vi "MMI GetAsyncKeyState.vi"(6 "Enum":T1(ring), 8 "error in (no error)":errorcluster) -> (0 "error out":errorcluster, 2 "Pressed?":bool, 5 "Pressed since last read?*":bool)   [LabVIEW 2021, in "Interaction By Refererence.lvclass"]
uses:
  Interaction By Refererence.lvclass
  user32.dll
panel:
  # "* This last read is OS global. If any other app reads GetAsyncKeyState, the value is reset!"
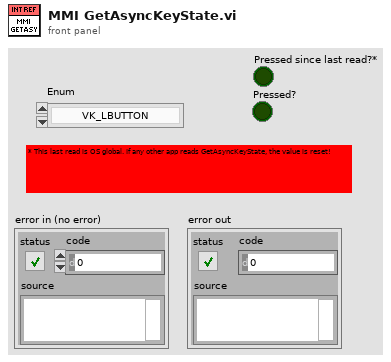
[diagram p1: front panel]
types:
  T1 = enum16{"VK_LBUTTON", "VK_RBUTTON", "VK_CANCEL", "VK_MBUTTON", "VK_XBUTTON1", "VK_XBUTTON2", "0x07", "VK_BACK", "VK_TAB", "0x0A", "0x0B", "VK_CLEAR", "VK_RETURN", "0x0E", "0x0F", "VK_SHIFT", "VK_CONTROL", "VK_MENU", "VK_PAUSE", "VK_CAPITAL", "VK_KANA\\VK_HANGUL", "0x16", "VK_JUNJA", "VK_FINAL", "VK_HANJA\\VK_KANJI", "0x1A", "VK_ESCAPE", "VK_CONVERT", "VK_NONCONVERT", "VK_ACCEPT", "VK_MODECHANGE", "VK_SPACE", "VK_PRIOR", "VK_NEXT", "VK_END", "VK_HOME", "VK_LEFT", "VK_UP", "VK_RIGHT", "VK_DOWN", "VK_SELECT", "VK_PRINT", "VK_EXECUTE", "VK_SNAPSHOT", "VK_INSERT", "VK_DELETE", "VK_HELP", "0 key", "1 key", "2 key", "3 key", "4 key", "5 key", "6 key", "7 key", "8 key", "9 key", "0x3A", "0x3B", "0x3C", "0x3D", "0x3E", "0x3F", "0x40", "A key", "B key", "C key", "D key", "E key", "F key", "G key", "H key", "I key", "J key", "K key", "L key", "M key", "N key", "O key", "P key", "Q key", "R key", "S key", "T key", "U key", "V key", "W key", "X key", "Y key", "Z key", "VK_LWIN", "VK_RWIN", "VK_APPS", "0x5E", "VK_SLEEP", "VK_NUMPAD0", "VK_NUMPAD1", "VK_NUMPAD2", "VK_NUMPAD3", "VK_NUMPAD4", "VK_NUMPAD5", "VK_NUMPAD6", "VK_NUMPAD7", "VK_NUMPAD8", "VK_NUMPAD9", "VK_MULTIPLY", "VK_ADD", "VK_SEPARATOR", "VK_SUBTRACT", "VK_DECIMAL", "VK_DIVIDE", "VK_F1", "VK_F2", "VK_F3", "VK_F4", "VK_F5", "VK_F6", "VK_F7", "VK_F8", "VK_F9", "VK_F10", "VK_F11", "VK_F12", "VK_F13", "VK_F14", "VK_F15", "VK_F16", "VK_F17", "VK_F18", "VK_F19", "VK_F20", "VK_F21", "VK_F22", "VK_F23", "VK_F24", "0x88", "0x89", "0x8A", "0x8B", "0x8C", "0x8D", "0x8E", "0x8F", "VK_NUMLOCK", "VK_SCROLL", "0x92", "0x93", "0x94", "0x95", "0x96", "0x97", "0x98", "0x99", "0x9A", "0x9B", "0x9C", "0x9D", "0x9E", "0x9F", "VK_LSHIFT", "VK_RSHIFT", "VK_LCONTROL", "VK_RCONTROL", "VK_LMENU", "VK_RMENU", "VK_BROWSER_BACK", "VK_BROWSER_FORWARD", "VK_BROWSER_REFRESH", "VK_BROWSER_STOP", "VK_BROWSER_SEARCH", "VK_BROWSER_FAVORITES", "VK_BROWSER_HOME", "VK_VOLUME_MUTE", "VK_VOLUME_DOWN", "VK_VOLUME_UP", "VK_MEDIA_NEXT_TRACK", "VK_MEDIA_PREV_TRACK", "VK_MEDIA_STOP", "VK_MEDIA_PLAY_PAUSE", "VK_LAUNCH_MAIL", "VK_LAUNCH_MEDIA_SELECT", "VK_LAUNCH_APP1", "VK_LAUNCH_APP2", "0xB8", "0xB9", "VK_OEM_1", "VK_OEM_PLUS", "VK_OEM_COMMA", "VK_OEM_MINUS", "VK_OEM_PERIOD", "VK_OEM_2", "VK_OEM_3", "0xC1", "0xC2", "0xC3", "0xC4", "0xC5", "0xC6", "0xC7", "0xC8", "0xC9", "0xCA", "0xCB", "0xCC", "0xCD", "0xCE", "0xCF", "0xD0", "0xD1", "0xD2", "0xD3", "0xD4", "0xD5", "0xD6", "0xD7", "0xD8", "0xD9", "0xDA", "VK_OEM_4", "VK_OEM_5", "VK_OEM_6", "VK_OEM_7", "VK_OEM_8", "0xE0", "0xE1", "VK_OEM_102", "0xE3", "0xE4", "VK_PROCESSKEY", "0xE6", "VK_PACKET", "0xE7", "0xE8", "0xE9", "0xEA", "0xEB", "0xEC", "0xED", "0xEF", "0xF0", "0xF1", "0xF2", "0xF3", "0xF4", "0xF5", "VK_ATTN", "VK_CRSEL", "VK_EXSEL", "VK_EREOF", "VK_PLAY", "VK_ZOOM", "VK_NONAME", "VK_PA1", "VK_OEM_CLEAR"}
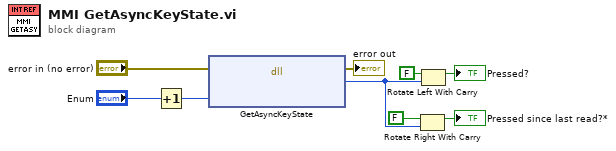
[diagram p0: block diagram]
diagram:
  n1 = Increment(x="Enum") -> (x+1=w1:T1)
  n2 = dll-call lib="user32.dll" fn="GetAsyncKeyState"(error in="error in (no error)", "x"=w1) -> (error out=→"error out":errorcluster, "return type"=w5:u16)  [unwired: 3 in, 1 out]
  n3 = Rotate Right With Carry(2:w5, 3:FALSE ("carry")) -> (1:→"Pressed since last read?*":bool)  [unwired: 1 out]
  n4 = Rotate Left With Carry(2:w5, 3:FALSE ("carry")) -> (1:→"Pressed?":bool)  [unwired: 1 out]
